vi "Kinematics_Begin.vi"   [LabVIEW 2020]
uses:
  Robot Global Data.vi
  <vilib>/Rock Robotics/WPI/ThirdParty/JAS_Junk/TrajLib/Trajectory_Library.lvlib
types:
  T1 = typedef "Trajectory_Library.lvlib/TRANSLATION2D.ctl" = cluster{"X":dbl, "Y":dbl}
  T2 = typedef "Trajectory_Library.lvlib/SWERVE_DRIVE_KINEMATICS.ctl" = cluster{"NumModules":i32, "InverseKinematics":T3, "ForwardKinematics":T3, "Modules":T1[], "PrevCoR":T1, "SavedModuleStates":T4[]}
  T3 = typedef "NI_Matrix.lvlib/RealMatrix.ctl" = dbl[][]
  T4 = typedef "Trajectory_Library.lvlib/SWERVE_DRIVE_MODULE_STATE.ctl" = cluster{"Speed":dbl, "Angle":T5}
  T5 = typedef "Trajectory_Library.lvlib/ROTATION2D.ctl" = cluster{"VALUE":dbl, "COS":dbl, "SIN":dbl}
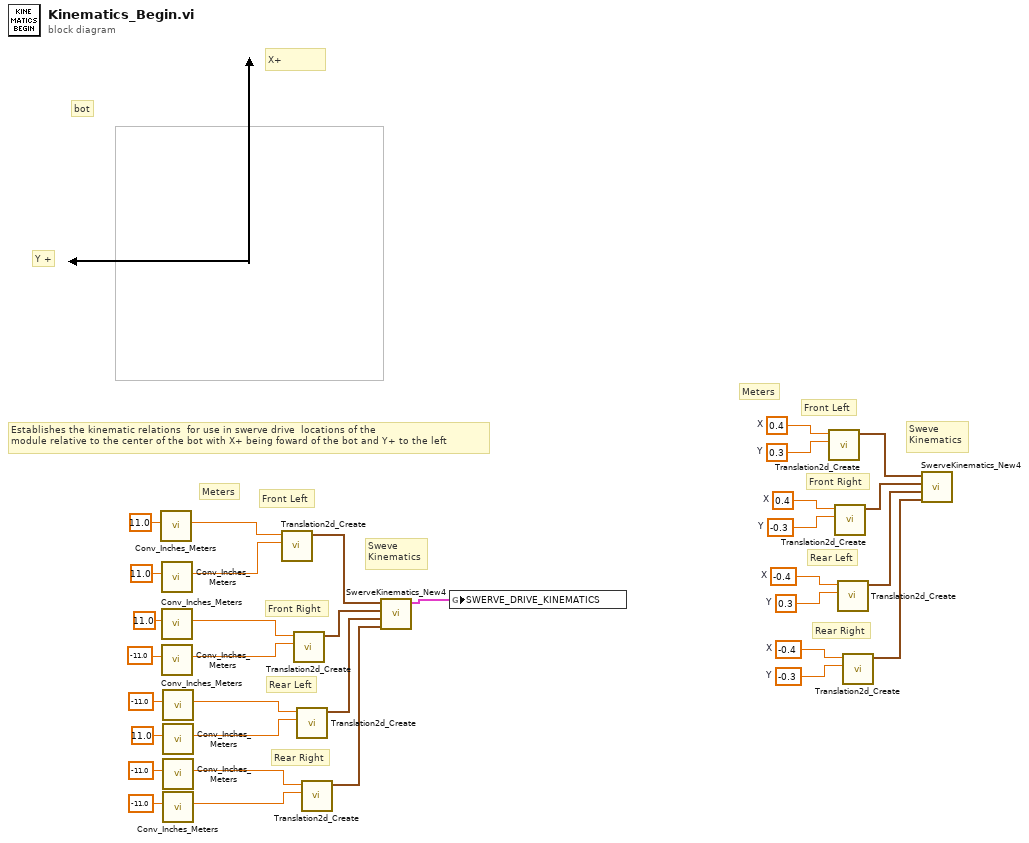
[diagram p0: block diagram]
diagram:
  w8 = -0.4  # X
  w7 = -0.3  # Y
  w6 = -0.4  # X
  w5 = 0.3  # Y
  w4 = 0.4  # X
  w3 = -0.3  # Y
  w2 = 0.4  # X
  w1 = 0.3  # Y
  # "Meters"
  # "Sweve\nKinematics"
  # "Rear Right"
  # "Rear Left"
  # "Front Right"
  # "Front Left"
  # "Establishes the kinematic relations  for use in swerve drive  locations of the \nmodule relative to the center of the bot with X+ being foward of the bot and Y+ to the left"
  # "Y +"
  # "X+"
  # "bot"
  # "Meters"
  # "Sweve\nKinematics"
  # "Rear Right"
  # "Rear Left"
  # "Front Right"
  # "Front Left"
  n1 = call <vilib>:"Conv_Inches_Meters.vi"("INCH"=11.0) -> ("Meters"=w19:dbl)  [unwired: 10 in]
  n2 = call <vilib>:"Conv_Inches_Meters.vi"("INCH"=11.0) -> ("Meters"=w27:dbl)  [unwired: 10 in]
  n3 = call <vilib>:"Conv_Inches_Meters.vi"("INCH"=11.0) -> ("Meters"=w18:dbl)  [unwired: 10 in]
  n4 = call <vilib>:"Conv_Inches_Meters.vi"("INCH"=-11.0) -> ("Meters"=w17:dbl)  [unwired: 10 in]
  n5 = call <vilib>:"Conv_Inches_Meters.vi"("INCH"=-11.0) -> ("Meters"=w16:dbl)  [unwired: 10 in]
  n6 = call <vilib>:"Conv_Inches_Meters.vi"("INCH"=11.0) -> ("Meters"=w15:dbl)  [unwired: 10 in]
  n7 = call <vilib>:"Conv_Inches_Meters.vi"("INCH"=-11.0) -> ("Meters"=w14:dbl)  [unwired: 10 in]
  n8 = call <vilib>:"Conv_Inches_Meters.vi"("INCH"=-11.0) -> ("Meters"=w13:dbl)  [unwired: 10 in]
  n9 = call <vilib>:"Translation2d_Create.vi"("Y"=w27, "X"=w19) -> ("TRANSLATION"=w30:T1)  [unwired: 9 in]
  n10 = call <vilib>:"Translation2d_Create.vi"("Y"=w17, "X"=w18) -> ("TRANSLATION"=w31:T1)  [unwired: 9 in]
  n11 = call <vilib>:"Translation2d_Create.vi"("Y"=w15, "X"=w16) -> ("TRANSLATION"=w32:T1)  [unwired: 9 in]
  n12 = call <vilib>:"Translation2d_Create.vi"("Y"=w13, "X"=w14) -> ("TRANSLATION"=w33:T1)  [unwired: 9 in]
  n13 = call <vilib>:"SwerveKinematics_New4.vi"("wheel 3"=w33, "wheel 2"=w32, "wheel 1"=w31, "wheel 0"=w30) -> ("SWERVE_DRIVE_KINEMATICS"=w29:T2)  [unwired: 7 in]
  n14 = global write "Robot Global Data.vi" "SWERVE_DRIVE_KINEMATICS"(w29) -> ()
  n15 = call <vilib>:"Translation2d_Create.vi"("Y"=w1, "X"=w2) -> ("TRANSLATION"=w9:T1)  [unwired: 9 in]
  n16 = call <vilib>:"Translation2d_Create.vi"("Y"=w3, "X"=w4) -> ("TRANSLATION"=w10:T1)  [unwired: 9 in]
  n17 = call <vilib>:"Translation2d_Create.vi"("Y"=w5, "X"=w6) -> ("TRANSLATION"=w11:T1)  [unwired: 9 in]
  n18 = call <vilib>:"Translation2d_Create.vi"("Y"=w7, "X"=w8) -> ("TRANSLATION"=w12:T1)  [unwired: 9 in]
  n19 = call <vilib>:"SwerveKinematics_New4.vi"("wheel 3"=w12, "wheel 2"=w11, "wheel 1"=w10, "wheel 0"=w9) -> ()  [unwired: 7 in, 1 out]
